vi "Array zusammenstutzen.vi"(6 "Speicher Freigeben":bool, 8 "Zeitstempeln":timestamp[](array[timestamp]), 10 "Anzahl Elemente":i32, 11 "Messdaten":sgl[][](array[numeric])) -> (0 "Zeitstempeln":timestamp[](array[timestamp]), 3 "Messdaten":sgl[][](array[numeric]))   [LabVIEW 2020, in "Messdaten.lvlib"]
uses:
  Messdaten.lvlib
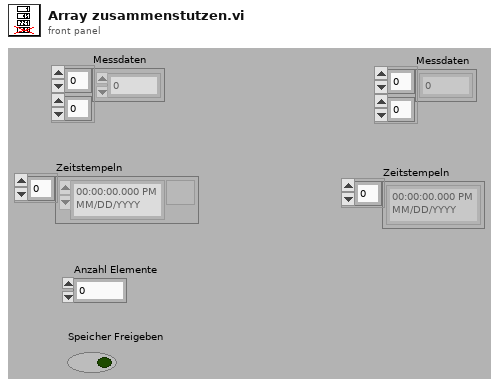
[diagram p1: front panel]
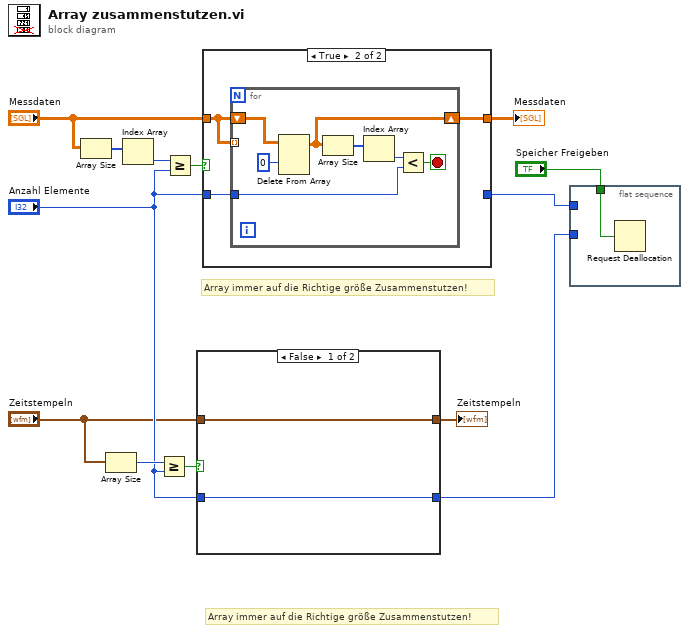
[diagram p0: block diagram]
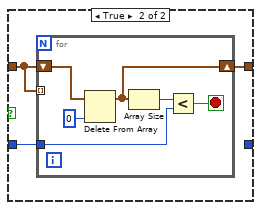
[diagram p2: hidden frame]
diagram:
  # "Array immer auf die Richtige größe Zusammenstutzen!"
  # "Array immer auf die Richtige größe Zusammenstutzen!"
  n1 = Array Size(array="Messdaten") -> (size(s)=w11:i32[])
  n2 = Array Size(array="Zeitstempeln") -> (size(s)=w7:i32)
  n3 = Index Array(array=w11) -> (element=w10:i32)  [unwired: 1 in]
  n4 = Greater Or Equal?(x=w7, y="Anzahl Elemente") -> (x >= y?=w9:bool)
  n5 = Greater Or Equal?(x=w10, y="Anzahl Elemente") -> (x >= y?=w13:bool)
  n6 = case shown="False" w9 {
    tunnel: "Zeitstempeln" -> [w15 w17]
    tunnel: [w15 w16] -> w4
    tunnel: "Anzahl Elemente" -> [w14 w18]
    tunnel: [w14 _] -> w2
    frame False {
    }
    frame True {
      n7 = for {
        tunnel: w18 -> [w22]
        tunnel: w17 -> [_] mode=indexing
        shift-right: [w19] -> w16
        shift-left: w17 -> [w24]
        stop <- w21 stop-if-true
        n8 = Delete From Array(array=w24, index=0 ("Index")) -> (array with subset deleted=w19:timestamp[])  [unwired: 1 in, 1 out]
        n9 = Array Size(array=w19) -> (size(s)=w23:i32)
        n10 = Less?(x=w23, y=w22) -> (x < y?=w21:bool)
      }
    }
  }
  "Zeitstempeln" <- w4
  n11 = case shown="True" w13 {
    tunnel: "Messdaten" -> [w26 w28]
    tunnel: [w26 w27] -> w8
    tunnel: "Anzahl Elemente" -> [w25 w29]
    tunnel: [w25 _] -> w3
    frame False {
    }
    frame True {
      n12 = for {
        tunnel: w29 -> [w35]
        tunnel: w28 -> [_] mode=indexing
        shift-right: [w32] -> w27
        shift-left: w28 -> [w36]
        stop <- w34 stop-if-true
        n13 = Delete From Array(array=w36, index (row)=0 ("Index")) -> (array with subset deleted=w32:sgl[][])  [unwired: 2 in, 1 out]
        n14 = Array Size(array=w32) -> (size(s)=w31:i32[])
        n15 = Index Array(array=w31) -> (element=w30:i32)  [unwired: 1 in]
        n16 = Less?(x=w30, y=w35) -> (x < y?=w34:bool)
      }
    }
  }
  "Messdaten" <- w8
  n17 = flat-sequence {
    tunnel: w3 -> [_]
    tunnel: w2 -> [_]
    tunnel: "Speicher Freigeben" -> [w37]
    frame #0 {
      n18 = Request Deallocation(w37) -> ()
    }
  }
